vi "Initialize.vi"(7 "thread ID":i32, 8 "error in (no error)":errorcluster, 9 "component name":string, 10 "Plugin Configuration":refnum<class "Plugin Configuration.lvclass">, 11 "UDPlog Transceiver in":refnum<class "UDPlog Transceiver.lvclass">) -> (0 "error out":errorcluster, 3 "UDPlog Transceiver out":refnum<class "UDPlog Transceiver.lvclass">)   [LabVIEW 2023, in "UDPlog.lvlib" / "UDPlog Transceiver.lvclass"]
uses:
  UDPlog Transceiver.lvclass
  Users/Public/Documents/National Instruments/NI VeriStand 2023/Custom Devices/Data Sharing Framework/Linux_x64/DSF Core.lvlibp/Classes/Configuration/Core/Plugin/Plugin Configuration.lvclass
  Users/Public/Documents/National Instruments/NI VeriStand 2023/Custom Devices/Data Sharing Framework/Linux_x64/DSF Core.lvlibp/Classes/Configuration/Core/Thread/Thread Configuration.lvclass
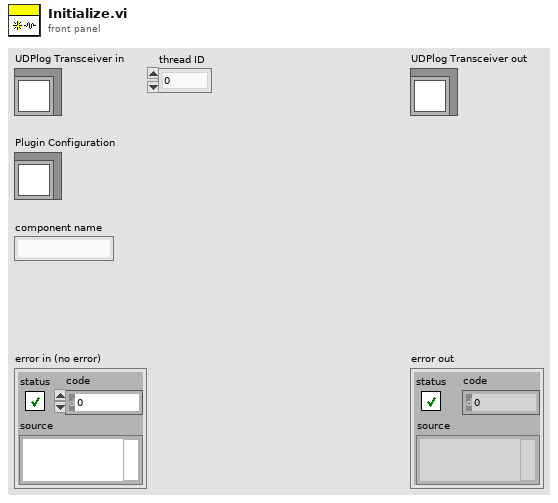
[diagram p1: front panel]
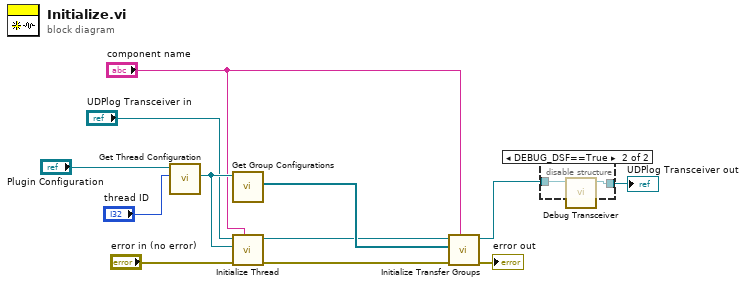
[diagram p0: block diagram]
diagram:
  n1 = call "Get Thread Configuration.vi"("index"="thread ID", "Plugin Configuration in"="Plugin Configuration") -> ("Thread Configuration"=w10:refnum<class "Thread Configuration.lvclass">)  [unwired: 7 in, 2 out]
  n2 = call "Get Group Configurations.vi"("Thread Configuration in"=w10) -> ("Group Configurations"=w4:refnum<class "Group Configuration.lvclass">[])  [unwired: 8 in, 2 out]
  n3 = call-dynamic "Initialize Thread.vi"("component name"="component name", "error in (no error)"="error in (no error)", "DSF Core.lvlibp:Thread Configuration.lvclass"=w10, "UDPlog Transceiver in"="UDPlog Transceiver in") -> ("error out"=w8:errorcluster, "UDPlog Transceiver out"=w1:refnum<class "UDPlog Transceiver.lvclass">)  [unwired: 6 in]
  n4 = call-dynamic "Initialize Transfer Groups.vi"("component name"="component name", "error in (no error)"=w8, "Group Configurations"=w4, "UDPlog Transceiver in"=w1) -> ("error out"=→"error out":errorcluster, "UDPlog Transceiver out"=w3:refnum<class "UDPlog Transceiver.lvclass">)  [unwired: 6 in]
  n5 = disable-structure shown="DEBUG_DSF==True" {
    disable-tunnel: w3 -> [w13 w15]
    disable-tunnel: [w13 w14] -> w2
    frame condition #0 (active) {
    }
    frame condition #1 {
      n6 = call "Debug Transceiver.vi"("UDPlog Transceiver in"=w15) -> ("UDPlog Transceiver out"=w14:refnum<class "UDPlog Transceiver.lvclass">)  [unwired: 10 in]
    }
  }
  "UDPlog Transceiver out" <- w2
